vi "Write Needle Valve.vi"(8 "error in (no error)":errorcluster, 10 "Heater":T1 max=100.0 scale=0.0..100.0 scale format="%.1f", 11 "Temperature Controller in":refnum<class "Temperature Controller.lvclass">) -> (0 "error out":errorcluster, 3 "Temperature Controller out":refnum<class "Temperature Controller.lvclass">)   [LabVIEW 2023, in "Temperature Controller.lvclass"]
uses:
  Temperature Controller.lvclass
  HV Slide Indicator.ctl
  Temperature Controller.lvclass/Temperature Controller.ctl
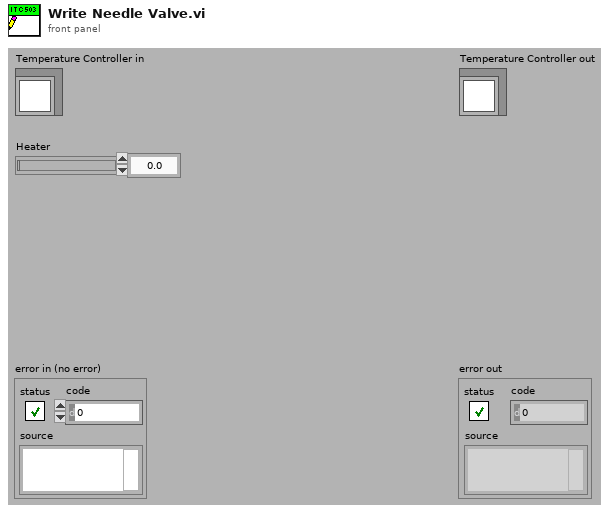
[diagram p1: front panel]
types:
  T1 = typedef "Temperature Controller.lvclass/HV Slide Indicator.ctl" = dbl
  T2 = typedef "ITCIO.ctl" = cluster{"Address":T3, "Version":T4, "Ch 1 dec places":i16, "Ch 2 dec places":i16, "Ch 3 dec places":i16, "Ch1 Name":string, "Ch2 Name":string, "Ch3 Name":string}
  T3 = typedef "OxfordAddress.ctl" = cluster{"Com Port":i32, "ISOBUS Address":i32, "GPIB Address":i16, "Communication":enum16{"RS232", "ISOBUS", "GPIB", "Gateway"}}
  T4 = typedef "ITCVersion.ctl" = enum16{"ITC502", "ITC503", "ITC601"}
  T5 = typedef "Temperature Controller.lvclass/AutoCtl.ctl" = cluster{"Auto Heater":bool, "Auto Needle":bool, "Auto PID":bool}
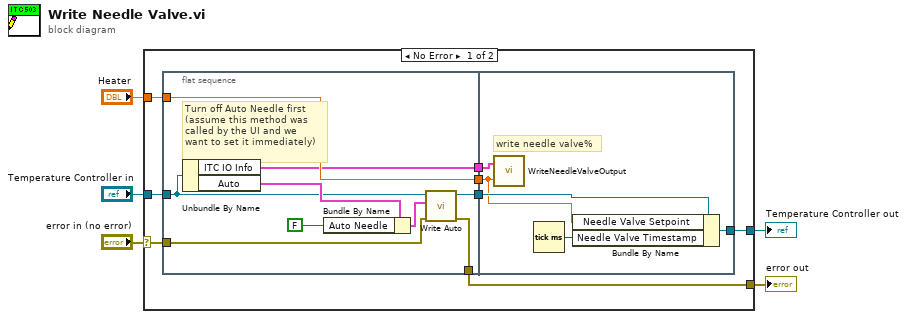
[diagram p0: block diagram]
diagram:
  n1 = case shown="No Error" "error in (no error)" {
    selector: "error in (no error)" -> [w8 w28]
    tunnel: [w7 w28] -> w4
    tunnel: [w12 w29] -> w2
    tunnel: "Temperature Controller in" -> [w13 w29]
    tunnel: "Heater" -> [w11 _]
    frame No Error {
      n2 = flat-sequence {
        tunnel: w11 -> [w22]
        tunnel: w13 -> [w19]
        tunnel: [w18] -> w10
        tunnel: [w22] -> w9
        tunnel: w8 -> [w17]
        tunnel: [w16] -> w7
        tunnel: [w14] -> w6
        tunnel: [w26] -> w12
        tunnel: w10 -> [w27]
        tunnel: w9 -> [w25]
        tunnel: w6 -> [w23]
        frame #0 {
          # "Turn off Auto Needle first\n(assume this method was\ncalled by the UI and we\nwant to set it immediately)"
          n3 = Unbundle By Name(w19) -> ("ITC IO Info"=w14:T2, "Auto"=w21:T5)
          n4 = Bundle By Name(cluster=w21, "Auto Needle"=FALSE) -> (w20:T5)
          n5 = call-dynamic "Write Auto.vi"("error in (no error)"=w17, "Auto"=w20, "Temperature Controller in"=w19) -> ("error out"=w16:errorcluster, "Temperature Controller out"=w18:refnum<class "Temperature Controller.lvclass">)  [unwired: 7 in]
        }
        frame #1 {
          # "write needle valve%"
          n6 = call "WriteNeedleValveOutput.vi"("Needle Valve Output (%"=w25, "ITC IO Info"=w23) -> ()  [unwired: 2 out]
          n7 = Tick Count (ms)() -> (millisecond timer value=w24:u32)
          n8 = Bundle By Name(cluster=w27, "Needle Valve Setpoint"=w25, "Needle Valve Timestamp"=w24) -> (w26:refnum<class "Temperature Controller.lvclass">)
        }
      }
    }
    frame Error {
    }
  }
  "error out" <- w4
  "Temperature Controller out" <- w2
